vi "myRIO v1.1 Open PWM.vi"(7 "Allow multiple opens?":bool, 8 "error in (no error)":errorcluster, 10 "Channel Name":string, 11 "Resource name":T1 caption="RIO Device") -> (0 "error out":errorcluster, 2 "PWM Channel":T2, 3 "myRIO Ref Out":T3)   [LabVIEW 2021]
uses:
  <vilib>/myRIO/Common/Instrument Driver Framework/Utilities/typedefs/myRIO v1.0 Reference.ctl
  <vilib>/myRIO/Common/Instrument Driver Framework/Utilities/typedefs/Generic FPGA Reference.ctl
  <vilib>/myRIO/Common/Instrument Driver Framework/myRIO v1.0/PWM/typedefs/PWM Channels Enum.ctl
  <vilib>/userDefined/High Color/nirio_resource_hc.ctl
  <vilib>/myRIO/Common/Instrument Driver Framework/myRIO v1.0/PWM/typedefs/myRIO v1.1 PWM Channels Enum.ctl
  <vilib>/myRIO/Common/Instrument Driver Framework/myRIO v1.0/PWM/vis/myRIO v1.0 Build MUX Configuration PWM.vi
  <vilib>/myRIO/Common/Instrument Driver Framework/myRIO v1.0/Resource Manager/vis/myRIO v1.0 Reserve Channel List.vi
  <vilib>/myRIO/Common/Instrument Driver Framework/myRIO v1.0/Resource Manager/vis/myRIO v1.0 Create Configuration List.vi
  <vilib>/myRIO/Common/Instrument Driver Framework/myRIO v1.0/Resource Manager/vis/myRIO v1.0 Reserve Channel.vi
  <vilib>/myRIO/Common/Instrument Driver Framework/myRIO v1.0/Resource Manager/vis/myRIO v1.0 Unreserve Channel.vi
  <vilib>/myRIO/Common/Instrument Driver Framework/myRIO v1.0/Resource Manager/vis/myRIO v1.0 Build Mutex Name.vi
  <vilib>/Utility/VariantDataType/GetNumericInfo.vi
  <vilib>/Utility/error.llb/Error Cluster From Error Code.vi
  <vilib>/myRIO/Common/Instrument Driver Framework/Utilities/vis/IO Manager.vi
  <vilib>/myRIO/Common/Instrument Driver Framework/Utilities/vis/Configuration Manager.vi
  <vilib>/myRIO/Common/Instrument Driver Framework/myRIO v1.0/Resource Manager/vis/myRIO v1.0 Configure IO.vi
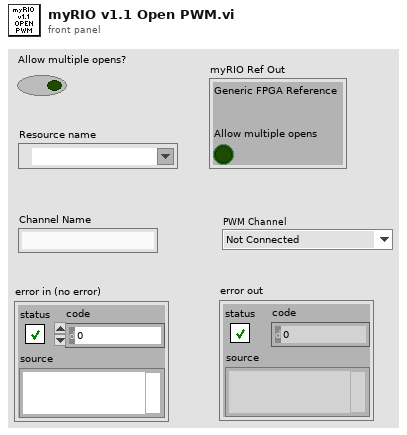
[diagram p1: front panel]
types:
  T1 = typedef "nirio_resource_hc.ctl" = tag
  T2 = typedef "PWM Channels Enum.ctl" = enum16{"Not Connected", "C/PWM0", "C/PWM1", "A/PWM0", "A/PWM1", "A/PWM2", "A/PWM3", "A/PWM4", "A/PWM5", "A/PWM6", "A/PWM7", "A/PWM8", "A/PWM9", "A/PWM10", "A/PWM11", "A/PWM12", "A/PWM13", "A/PWM14", "A/PWM15", "A/PWM16", "A/PWM17", "A/PWM18", "A/PWM19", "B/PWM0", "B/PWM1", "B/PWM2", "B/PWM3", "B/PWM4", "B/PWM5", "B/PWM6", "B/PWM7", "B/PWM8", "B/PWM9", "B/PWM10", "B/PWM11", "B/PWM12", "B/PWM13", "B/PWM14", "B/PWM15", "B/PWM16", "B/PWM17", "B/PWM18", "B/PWM19", "PWM/PWM0", "PWM/PWM1", "PWM/PWM2", "PWM/PWM3", "PWM/PWM4", "PWM/PWM5", "PWM/PWM6", "PWM/PWM7", "PWM/PWM8", "PWM/PWM9"}
  T3 = typedef "myRIO v1.0 Reference.ctl" = cluster{"Generic FPGA Reference":T4, "Allow multiple opens":bool}
  T4 = typedef "Generic FPGA Reference.ctl" = refnum<k20>
  T5 = typedef "myRIO v1.1 PWM Channels Enum.ctl" = enum16{"Not Connected", "C/PWM0", "C/PWM1", "A/PWM0", "A/PWM1", "A/PWM2", "B/PWM0", "B/PWM1", "B/PWM2"}
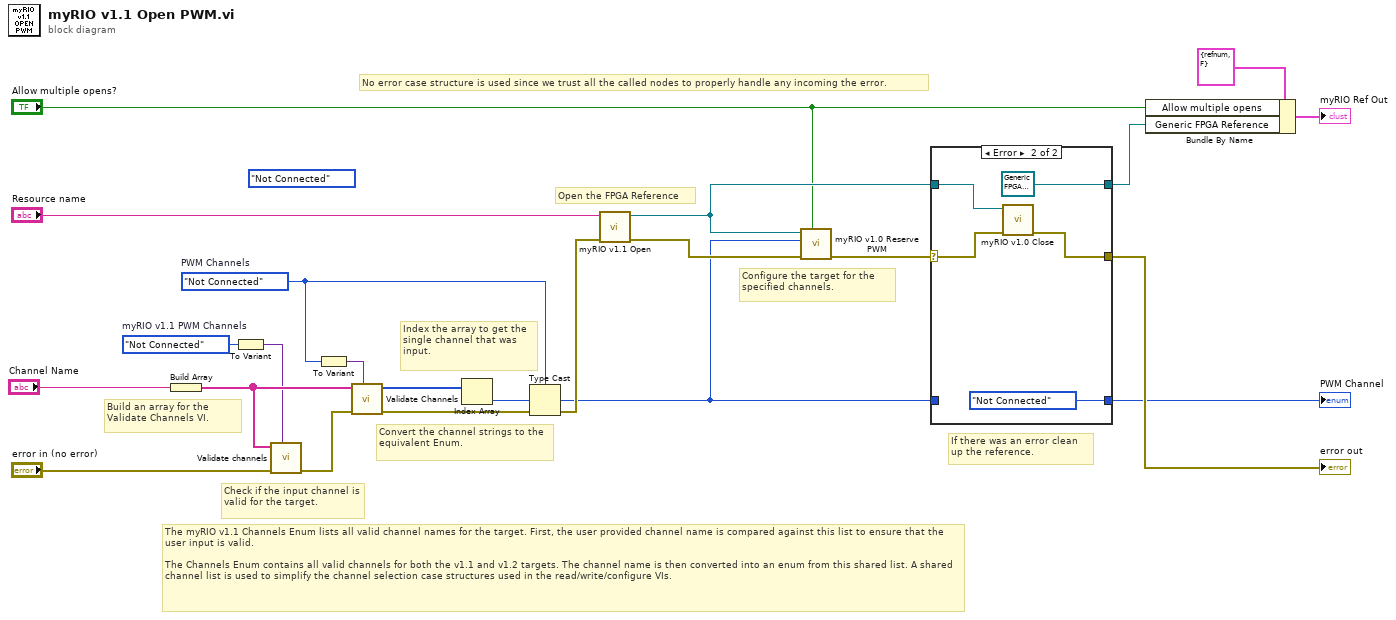
[diagram p0: block diagram]
diagram:
  (unwired) PWM_Channels_Enum."Not Connected" ("PWM Channels Enum")
  w2 = myRIO_v1.1_PWM_Channels_Enum."Not Connected"  # myRIO v1.1 PWM Channels
  w1 = PWM_Channels_Enum."Not Connected"  # PWM Channels
  # "The myRIO v1.1 Channels Enum lists all valid channel names for the target. First, the user provided channel name is compared against this list to ensure that the user input is valid.\n\nThe Channels Enum contains all valid channels for both the v1.1 and v1.2 targets. The channel name is then converted into an enum from this shared list. A shared channel list is used to simplify the channel selection case structures used in the read/write/configure VIs."
  # "Index the array to get the single channel that was input."
  # "Build an array for the Validate Channels VI."
  # "If there was an error clean up the reference."
  # "Configure the target for the specified channels."
  # "Open the FPGA Reference"
  # "No error case structure is used since we trust all the called nodes to properly handle any incoming the error."
  # "Convert the channel strings to the equivalent Enum."
  # "Check if the input channel is valid for the target."
  n1 = Build Array("Channel Name") -> (w12:string[])
  n2 = To Variant(anything=w2) -> (Variant=w3:variant)
  n3 = call <vilib>:"Validate channels.vi"("Channels Enum Variant"=w3, "error in (no error)"="error in (no error)", "Channel Names"=w12) -> ("error out"=w21:errorcluster)  [unwired: 7 in, 1 out]
  n4 = To Variant(anything=w1) -> (Variant=w4:variant)
  n5 = call <vilib>:"Validate Channels.vi"("Channels Enum Variant"=w4, "error in (no error)"=w21, "Channel Names"=w12) -> ("error out"=w17:errorcluster, "Index Array"=w11:u16[])  [unwired: 7 in]
  n6 = Index Array(array=w11) -> (element=w10:u16)  [unwired: 1 in]
  n7 = Type Cast(type=w1, x=w10) -> (*(type *) &x=w9:T2)
  n8 = call <vilib>:"myRIO v1.1 Open.vi"("error in (no error)"=w17, "Resource name"="Resource name") -> ("error out"=w16:errorcluster, "myRIO FPGA Ref Out"=w14:T4)  [unwired: 8 in]
  n9 = call <vilib>:"myRIO v1.0 Reserve PWM.vi"("Allow multiple opens?"="Allow multiple opens?", "error in (no error)"=w16, "PWM Channel"=w9, "myRIO FPGA Ref Out"=w14) -> ("error out"=w15:errorcluster)  [unwired: 7 in]
  n10 = case shown="Error" w15 {
    selector: w15 -> [w24 w30]
    tunnel: w14 -> [w25 w28]
    tunnel: [w25 T4 refnum ("myRIO FPGA Ref Out")] -> w19
    tunnel: [w24 w29] -> w18
    tunnel: w9 -> [w23 _]
    tunnel: [w23 PWM_Channels_Enum."Not Connected"] -> w8
    frame No Error {
    }
    frame Error {
      n11 = call <vilib>:"myRIO v1.0 Close.vi"("error in (no error)"=w30, "myRIO FPGA Ref In"=w28) -> ("error out"=w29:errorcluster)  [unwired: 9 in]
    }
  }
  "PWM Channel" <- w8
  "error out" <- w18
  n12 = Bundle By Name(cluster=T3 {"Generic FPGA Reference"=refnum, "Allow multiple opens"=FALSE} ("myRIO v1.0 Reference"), "Allow multiple opens"="Allow multiple opens?", "Generic FPGA Reference"=w19) -> (→"myRIO Ref Out":T3)
